vi "Method Name Validation.vi"(10 "Methods List in":string[](array[string]), 11 "Method Name in":string) -> (2 "Validation Status out":bool, 3 "Log Message out":string)   [LabVIEW 2013, in "Scripter.lvlib"]
uses:
  Scripter.lvlib
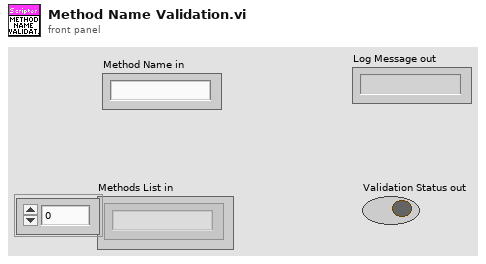
[diagram p1: front panel]
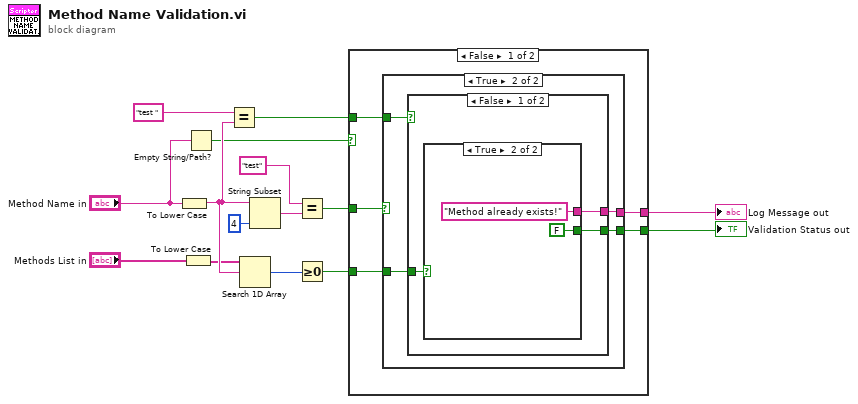
[diagram p0: block diagram]
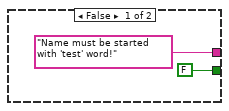
[diagram p2: hidden frame]
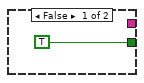
[diagram p3: hidden frame]
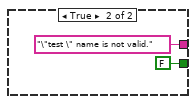
[diagram p4: hidden frame]
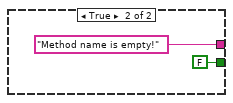
[diagram p5: hidden frame]
diagram:
  n1 = To Lower Case(string="Method Name in") -> (all lower case string=w14:string)
  n2 = To Lower Case(string="Methods List in") -> (all lower case string=w9:string[])
  n3 = Empty String/Path?(string/path="Method Name in") -> (empty?=w13:bool)
  n4 = Equal?(x="test " ("New Test Method Name"), y=w14) -> (x = y?=w1:bool)
  n5 = Search 1D Array(1D array=w9, element=w14) -> (index of element=w10:i32)  [unwired: 1 in]
  n6 = String Subset(string=w14, length (rest)=4 ("length (rest)")) -> (substring=w3:string)  [unwired: 1 in]
  n7 = Equal?(x="test", y=w3) -> (x = y?=w5:bool)
  n8 = Greater Or Equal To 0?(x=w10) -> (x >= 0?=w11:bool)
  n9 = case shown="False" w13 {
    tunnel: w5 -> [w20 _]
    tunnel: [w19 "Method name is empty!"] -> w6
    tunnel: [w18 FALSE] -> w7
    tunnel: w11 -> [w17 _]
    tunnel: w1 -> [w16 _]
    frame False {
      n10 = case shown="True" w20 {
        tunnel: ["Name must be started with 'test' word!" w24] -> w19
        tunnel: [FALSE w26] -> w18
        tunnel: w17 -> [_ w25]
        tunnel: w16 -> [_ w23]
        frame False {
        }
        frame True {
          n11 = case shown="False" w23 {
            tunnel: [w29 FALSE] -> w26
            tunnel: w25 -> [w28 _]
            tunnel: [w27 "\"test \" name is not valid."] -> w24
            frame False {
              n12 = case shown="True" w28 {
                tunnel: [TRUE FALSE] -> w29
                tunnel: [_ "Method already exists!"] -> w27
                frame False {
                }
                frame True {
                }
              }
            }
            frame True {
            }
          }
        }
      }
    }
    frame True {
    }
  }
  "Validation Status out" <- w7
  "Log Message out" <- w6
